vi "Resistance Test_BU3.vi"(0 "DMM ref in":refnum<visa-resource-name>, 2 "Resistance Test REF":refnum<vi>, 3 "Resistance Test Stop REF":refnum<vi>, 5 "DMM error in":errorcluster, 7 "Channel  Count":i32, 9 "ESP32 ref in":refnum<visa-resource-name>="COM4", 11 "ESP32 error in":errorcluster, 12 "Wait Current Stable Period":u32, 14 "Current Sense \nResitance Array":dbl[](array[numeric])) -> (1 "Array 2":bool[](array[boolean]), 6 "error?":bool, 8 "Array":dbl[](array[numeric]), 10 "ESP32 ref out":refnum<visa-resource-name>, 15 "ESP32 error out":errorcluster)   [LabVIEW 2023]
uses:
  <instrlib>/Agilent 3446X Series/Agilent 3446X Series.lvlib
panel:
  out "Array 3":i32[][](array[numeric])
  out "error? 2":bool
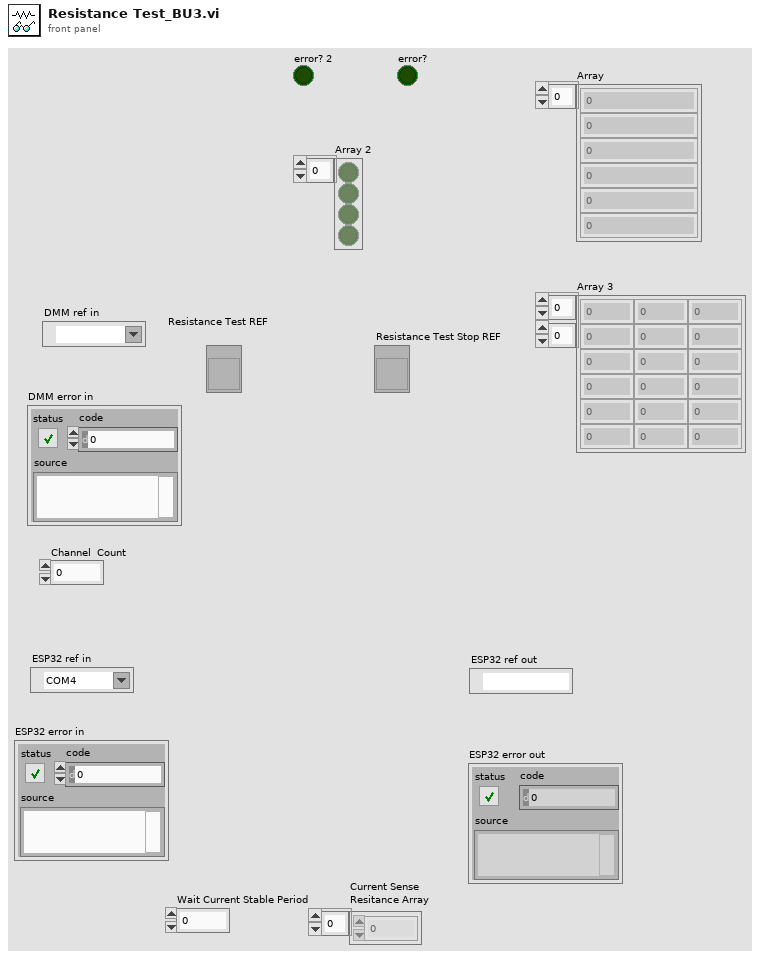
[diagram p1: front panel]
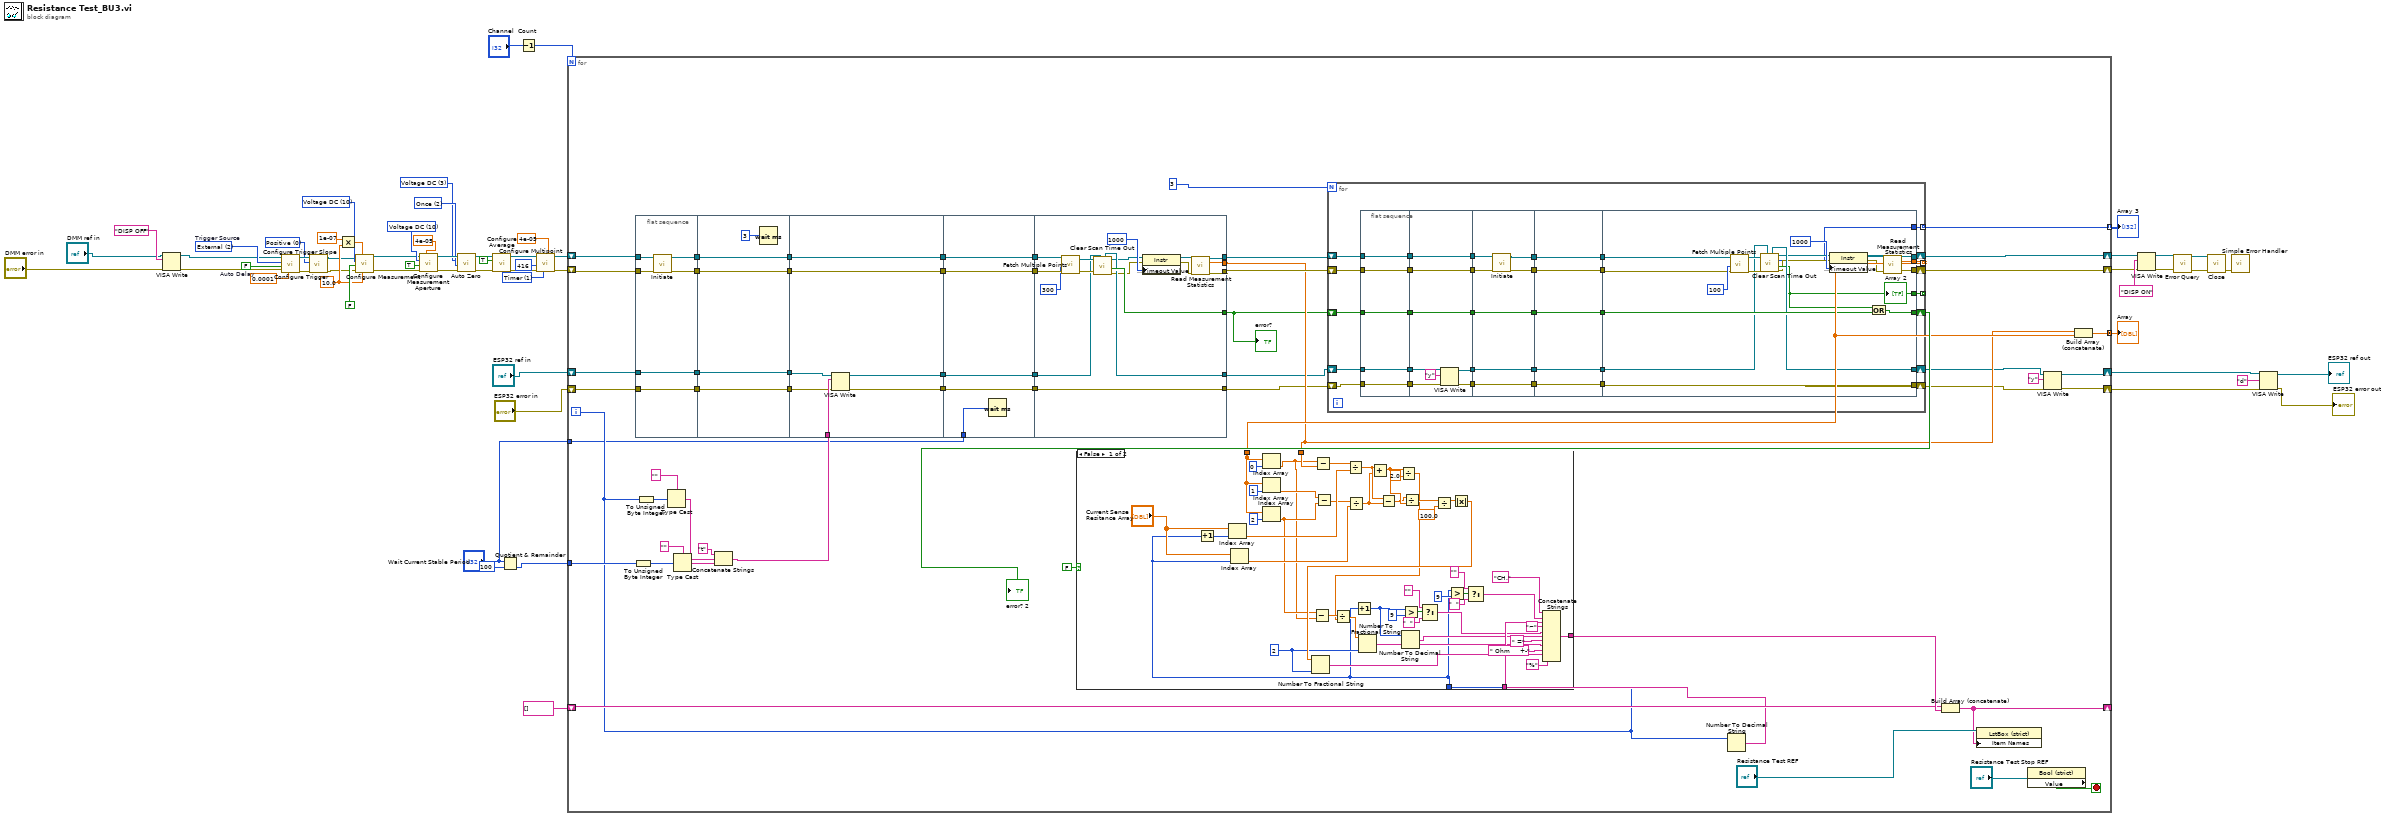
[diagram p0: block diagram]
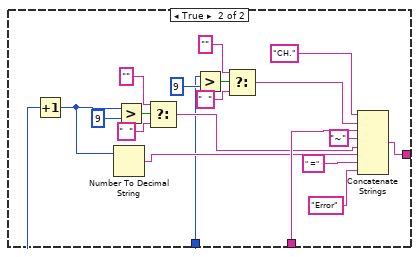
[diagram p2: hidden frame]
diagram:
  w20 = 0 items=["Positive", "Negative"] ("Trigger Edge (1: Negative)")
  w18 = 2 items=["Immediate", "Software (Bus)", "External"]  # Trigger Source
  w19 = FALSE  # Auto Delay
  w23 = 10.0 ("Manual Range (1)")
  w27 = 10 items=["Continuity", "Current AC", "Current DC", "Diode", "Frequency", "Resistance 4-wire", "Period", "Resistance 2-wire", "Temperature", "Voltage AC", "Voltage DC", "Voltage DC Ratio", "Capacitance"] ("Measurement Function (10: Voltage DC)")
  w31 = 1 items=["Immediate", "Timer"] ("Sample Source (0: Immediate)")
  w38 = 3 items=["Current DC", "Resistance", "Temperature", "Voltage DC"] ("Zero Type (0: Current DC)")
  w39 = 2 items=["Disable", "Enable", "Once"] ("Auto Zero (1: Enable)")
  w35 = 10 items=["Continuity", "Current AC", "Current DC", "Diode", "Frequency", "Resistance 4-wire", "Period", "Resistance 2-wire", "Temperature", "Voltage AC", "Voltage DC", "Voltage DC Ratio", "Capacitance"] ("Measurement Function (0: Continuity)")
  n1 = VISA Write(VISA resource name="DMM ref in", write buffer="DISP OFF", error in (no error)="DMM error in") -> (VISA resource name out=w2:refnum<visa-resource-name>, error out=w1:errorcluster)  [unwired: 1 out]
  n2 = call <instrlib>:"Configure Trigger.vi"("Manual Trigger Delay (1 s)"=0.0001, "error in (no error)"=w1, "Auto Delay (F:Disable)"=w19, "Trigger Source (0: Immediate)"=w18, "VISA resource name"=w2) -> ("error out"=w22:errorcluster, "VISA resource name out"=w21:refnum<visa-resource-name>)  [unwired: 1 in, 4 out]
  n3 = call <instrlib>:"Configure Trigger Slope.vi"("error in (no error)"=w22, "Trigger Edge (1: Negative)"=w20, "VISA resource name"=w21) -> ("error out"=w15:errorcluster, "VISA resource name out"=w16:refnum<visa-resource-name>)  [unwired: 7 in]
  n4 = Multiply(x=1e-07, y=w23) -> (x*y=w28:dbl)
  n5 = call <instrlib>:"Configure Measurement.vi"("Manual Range (1)"=w23, "Absolute Resolution (1E-6)"=w28, "error in (no error)"=w15, "Auto Range (T: Enable)"=FALSE, "Measurement Function (10: Voltage DC)"=w27, "VISA resource name"=w16) -> ("error out"=w24:errorcluster, "VISA resource name out"=w25:refnum<visa-resource-name>)  [unwired: 4 out]
  n6 = call <instrlib>:"Configure Measurement Aperture.vi"("Aperture Time (0.1s)"=4e-05, "error in (no error)"=w24, "Enable Aperture (F: Disable)"=TRUE, "Measurement Function (0: Continuity)"=w35, "VISA resource name"=w25) -> ("error out"=w42:errorcluster, "VISA resource name out"=w41:refnum<visa-resource-name>)  [unwired: 5 in]
  n7 = call <instrlib>:"Auto Zero.vi"("error in (no error)"=w42, "Auto Zero (1: Enable)"=w39, "Zero Type (0: Current DC)"=w38, "VISA resource name"=w41) -> ("error out"=w44:errorcluster, "VISA resource name out"=w43:refnum<visa-resource-name>)  [unwired: 6 in]
  n8 = call <instrlib>:"Configure Average.vi"("error in (no error)"=w44, "Enable Statistics (F: Disable)"=TRUE, "VISA resource name"=w43) -> ("error out"=w33:errorcluster, "VISA resource name out"=w34:refnum<visa-resource-name>)  [unwired: 7 in]
  n9 = Quotient & Remainder(x="Wait Current Stable Period", y=100) -> (floor(x/y)=w11:u32)  [unwired: 1 out]
  n10 = Decrement(x="Channel  Count") -> (x-1=w9:i32)
  n11 = call <instrlib>:"Configure Multipoint.vi"("Sample Interval (1 Second)"=4e-05, "Sample Source (0: Immediate)"=w31, "error in (no error)"=w33, "Sample Count (1)"=416, "VISA resource name"=w34) -> ("error out"=w13:errorcluster, "VISA resource name out"=w14:refnum<visa-resource-name>)  [unwired: 2 in, 3 out]
  n12 = for {
    N: w9 -> [_]
    shift-right: [w65] -> w46
    shift-left: "ESP32 ref in" -> [w100]
    shift-right: [w63] -> w10
    shift-left: "ESP32 error in" -> [w98]
    shift-right: [w110] -> w47
    shift-left: w13 -> [w104]
    shift-right: [w111] -> w48
    shift-left: w14 -> [w105]
    shift-right: [w113] -> _
    shift-left: string[] [] -> [w115]
    tunnel: w11 -> [w88]
    tunnel: [w81] -> w8 mode=concatenating
    tunnel: "Wait Current Stable Period" -> [w69]
    tunnel: [w61] -> w6 mode=indexing
    i -> [w85]
    stop <- w117 stop-if-true
    n13 = To Unsigned Byte Integer(number=w88) -> (unsigned 8bit integer=w92:u8)
    n14 = flat-sequence {
      tunnel: w104 -> [w190]
      tunnel: w105 -> [w192]
      tunnel: [w191] -> w109
      tunnel: [w189] -> w108
      tunnel: [w188] -> w101
      tunnel: w100 -> [w188]
      tunnel: w98 -> [w187]
      tunnel: [w187] -> w97
      tunnel: [w197] -> w107
      tunnel: [w196] -> w106
      tunnel: w109 -> [w197]
      tunnel: w108 -> [w196]
      tunnel: w101 -> [w194]
      tunnel: [w194] -> w99
      tunnel: w97 -> [w193]
      tunnel: [w193] -> w96
      tunnel: w107 -> [w204]
      tunnel: [w204] -> w75
      tunnel: w106 -> [w203]
      tunnel: [w203] -> w77
      tunnel: w99 -> [w202]
      tunnel: w96 -> [w200]
      tunnel: w87 -> [w201]
      tunnel: [w199] -> w73
      tunnel: [w198] -> w71
      tunnel: w77 -> [w209]
      tunnel: [w209] -> w76
      tunnel: w75 -> [w208]
      tunnel: [w208] -> w74
      tunnel: w73 -> [w207]
      tunnel: [w207] -> w72
      tunnel: w71 -> [w206]
      tunnel: [w206] -> w70
      tunnel: w69 -> [w205]
      tunnel: [w223] -> w102
      tunnel: [w224] -> w103
      tunnel: w76 -> [w226]
      tunnel: w74 -> [w225]
      tunnel: [w215] -> w78
      tunnel: w72 -> [w217]
      tunnel: [w221] -> w68
      tunnel: w70 -> [w221]
      tunnel: [w220] -> w82
      tunnel: [w216] -> w79
      frame #0 {
        n15 = call <instrlib>:"Initiate.vi"("error in (no error)"=w190, "VISA resource name"=w192) -> ("error out"=w189:errorcluster, "VISA resource name out"=w191:refnum<visa-resource-name>)  [unwired: 8 out]
      }
      frame #1 {
        n16 = Wait (ms)(milliseconds to wait=u32 3) -> ()  [unwired: 1 out]
      }
      frame #2 {
        n17 = VISA Write(VISA resource name=w202, write buffer=w201, error in (no error)=w200) -> (VISA resource name out=w199:refnum<visa-resource-name>, error out=w198:errorcluster)  [unwired: 1 out]
      }
      frame #3 {
        n18 = Wait (ms)(milliseconds to wait=w205) -> ()  [unwired: 1 out]
      }
      frame #4 {
        n19 = call <instrlib>:"Fetch Multiple Points.vi"("error in (no error)"=w226, "Timeout (10000 ms)"=300, "VISA resource name"=w225) -> ("error out"=w218:errorcluster, "VISA resource name out"=w219:refnum<visa-resource-name>)  [unwired: 1 in, 6 out]
        n20 = call "Clear Scan Time Out.vi"("ESP32 ref"=w217, "error in (no error)"=w218, "VISA Refnum in"=w219) -> ("error out"=w212:errorcluster, "error?"=w216:bool, "VISA Refnum out"=w213:refnum<visa-resource-name>, "ESP32 ref out"=w215:refnum<visa-resource-name>)  [unwired: 4 in, 1 out]
        n21 = property class="Instr"(reference=w213, error in=w212, "General Settings:Timeout Value"=u32 1000) -> (reference out=w211:refnum<visa-resource-name>, error out=w210:errorcluster)
        n22 = call <instrlib>:"Read Measurement Statistics.vi"("VISA resource name"=w211, "error in (no error)"=w210) -> ("VISA resource name out"=w224:refnum<visa-resource-name>, "Arithmetic Mean"=w220:dbl, "error out"=w223:errorcluster)  [unwired: 6 in, 5 out]
      }
    }
    n23 = To Unsigned Byte Integer(number=w85) -> (unsigned 8bit integer=w89:u8)
    n24 = Type Cast(type="" ("string"), x=w89) -> (*(type *) &x=w90:string)
    n25 = Type Cast(type="" ("string"), x=w92) -> (*(type *) &x=w91:string)
    n26 = Concatenate Strings("t" ("data in"), w90, w91) -> (w87:string)
    n27 = for {
      N: 3 -> [_]
      tunnel: [w257] -> w83 mode=indexing
      shift-right: [w256] -> w111
      shift-left: w103 -> [w259]
      shift-right: [w255] -> w110
      shift-left: w102 -> [w258]
      shift-right: [w253] -> w84
      shift-left: w79 -> [w254]
      tunnel: [w250] -> w80 mode=indexing
      shift-right: [w251] -> w66
      shift-left: w78 -> [w252]
      shift-right: [w248] -> w64
      shift-left: w68 -> [w249]
      tunnel: [w247] -> w61 mode=indexing
      n28 = flat-sequence {
        tunnel: w249 -> [w260]
        tunnel: w252 -> [w261]
        tunnel: w254 -> [w262]
        tunnel: w258 -> [w263]
        tunnel: w259 -> [w264]
        tunnel: [w264] -> w246
        tunnel: [w263] -> w245
        tunnel: [w262] -> w244
        tunnel: [w261] -> w243
        tunnel: [w260] -> w242
        tunnel: [w272] -> w241
        tunnel: [w271] -> w240
        tunnel: [w270] -> w239
        tunnel: [w268] -> w238
        tunnel: [w265] -> w237
        tunnel: w246 -> [w272]
        tunnel: w245 -> [w271]
        tunnel: w244 -> [w270]
        tunnel: w243 -> [w269]
        tunnel: w242 -> [w266]
        tunnel: w241 -> [w276]
        tunnel: w240 -> [w275]
        tunnel: [w274] -> w236
        tunnel: w239 -> [w279]
        tunnel: [w279] -> w234
        tunnel: w238 -> [w278]
        tunnel: [w278] -> w232
        tunnel: w237 -> [w277]
        tunnel: [w277] -> w230
        tunnel: [w273] -> w228
        tunnel: w236 -> [w284]
        tunnel: [w284] -> w235
        tunnel: w234 -> [w283]
        tunnel: [w283] -> w233
        tunnel: w232 -> [w282]
        tunnel: [w282] -> w231
        tunnel: w230 -> [w281]
        tunnel: [w281] -> w229
        tunnel: w228 -> [w280]
        tunnel: [w280] -> w227
        tunnel: [w304] -> w257
        tunnel: [w302] -> w256
        tunnel: [w301] -> w255
        tunnel: [w299] -> w253
        tunnel: [w295] -> w251
        tunnel: [w294] -> w250
        tunnel: w235 -> [w285]
        tunnel: w233 -> [w300]
        tunnel: w231 -> [w296]
        tunnel: w229 -> [w288]
        tunnel: [w288] -> w248
        tunnel: [w287] -> w247
        tunnel: w227 -> [w286]
        frame #0 {
        }
        frame #1 {
          n29 = VISA Write(VISA resource name=w269, write buffer="y", error in (no error)=w266) -> (VISA resource name out=w268:refnum<visa-resource-name>, error out=w265:errorcluster)  [unwired: 1 out]
        }
        frame #2 {
          n30 = call <instrlib>:"Initiate.vi"("error in (no error)"=w275, "VISA resource name"=w276) -> ("error out"=w274:errorcluster, "VISA resource name out"=w273:refnum<visa-resource-name>)  [unwired: 8 out]
        }
        frame #3 {
        }
        frame #4 {
          n31 = call <instrlib>:"Fetch Multiple Points.vi"("error in (no error)"=w285, "Timeout (10000 ms)"=100, "VISA resource name"=w286) -> ("error out"=w297:errorcluster, "VISA resource name out"=w298:refnum<visa-resource-name>)  [unwired: 1 in, 6 out]
          n32 = call "Clear Scan Time Out.vi"("ESP32 ref"=w296, "error in (no error)"=w297, "VISA Refnum in"=w298) -> ("error out"=w289:errorcluster, "error?"=w294:bool, "Time out count"=w287:i32, "VISA Refnum out"=w290:refnum<visa-resource-name>, "ESP32 ref out"=w295:refnum<visa-resource-name>)  [unwired: 4 in]
          n33 = property class="Instr"(reference=w290, error in=w289, "General Settings:Timeout Value"=u32 1000) -> (reference out=w292:refnum<visa-resource-name>, error out=w291:errorcluster)
          n34 = Or(x=w294, y=w300) -> (x .or. y?=w299:bool)
          n35 = call <instrlib>:"Read Measurement Statistics.vi"("VISA resource name"=w292, "error in (no error)"=w291) -> ("VISA resource name out"=w302:refnum<visa-resource-name>, "Arithmetic Mean"=w304:dbl, "error out"=w301:errorcluster)  [unwired: 6 in, 5 out]
        }
      }
    }
    "Array 2" <- w80
    "error? 2" <- w84
    n36 = Number To Decimal String(number=w85) -> (decimal integer string=w86:string)  [unwired: 1 in]
    n37 = case shown="False" FALSE {
      tunnel: [w162 w181] -> w116
      tunnel: w86 -> [w159 w178]
      tunnel: w83 -> [w147 _]
      tunnel: w85 -> [w123 w169]
      tunnel: w82 -> [w140 _]
      frame False {
        w131 = i16 2 ("precision (6)")
        n38 = Increment(x=w123) -> (x+1=w143:i32)
        n39 = Index Array(array="Current Sense \nResitance Array", index=w143) -> (element=w141:dbl)
        n40 = Index Array(array="Current Sense \nResitance Array", index=w123) -> (element=w138:dbl)
        n41 = Index Array(array=w147, index=0) -> (element=w127:dbl)
        n42 = Index Array(array=w147, index=1) -> (element=w128:dbl)
        n43 = Index Array(array=w147, index=2) -> (element=w129:dbl)
        n44 = Subtract(x=w129, y=w127) -> (x-y=w126:dbl)
        n45 = Subtract(x=w127, y=w140) -> (x-y=w144:dbl)
        n46 = Subtract(x=w128, y=w129) -> (x-y=w139:dbl)
        n47 = Divide(x=w144, y=w141) -> (x/y=w136:dbl)
        n48 = Divide(x=w139, y=w138) -> (x/y=w135:dbl)
        n49 = Increment(x=w123) -> (x+1=w152:i32)
        n50 = Add(x=w136, y=w135) -> (x+y=w122:dbl)
        n51 = Subtract(x=w136, y=w135) -> (x-y=w121:dbl)
        n52 = Divide(x=w122, y=2.0) -> (x/y=w125:dbl)
        n53 = Divide(x=w126, y=w125) -> (x/y=w124:dbl)
        n54 = Number To Fractional String(number=w124, precision (6)=w131) -> (F-format string=w133:string)  [unwired: 2 in]
        n55 = Number To Decimal String(number=w152) -> (decimal integer string=w151:string)  [unwired: 1 in]
        n56 = Greater?(x=w152, y=9) -> (0:w156:bool)
        n57 = Divide(x=w121, y=w122) -> (x/y=w134:dbl)
        n58 = Select(t="" ("string"), s=w156, f="  " ("string")) -> (s? t:f=w153:string)
        n59 = Divide(x=w134, y=100.0) -> (x/y=w120:dbl)
        n60 = Greater?(x=w123, y=9) -> (0:w165:bool)
        n61 = Absolute Value(x=w120) -> (abs(x)=w132:dbl)
        n62 = Number To Fractional String(number=w132, precision (6)=w131) -> (F-format string=w130:string)  [unwired: 2 in]
        n63 = Select(t="" ("string"), s=w165, f="  " ("string")) -> (s? t:f=w160:string)
        n64 = Concatenate Strings("CH." ("string"), w160, w159, "~" ("string"), w153, w151, " =" ("string"), w133, " Ohm     +-" ("string"), w130, "%" ("string")) -> (w162:string)
      }
      frame True {
        n65 = Increment(x=w169) -> (x+1=w171:i32)
        n66 = Number To Decimal String(number=w171) -> (decimal integer string=w170:string)  [unwired: 1 in]
        n67 = Greater?(x=w171, y=9) -> (0:w175:bool)
        n68 = Select(t="" ("string"), s=w175, f="  " ("string")) -> (s? t:f=w172:string)
        n69 = Greater?(x=w169, y=9) -> (0:w184:bool)
        n70 = Select(t="" ("string"), s=w184, f="  " ("string")) -> (s? t:f=w179:string)
        n71 = Concatenate Strings("CH." ("string"), w179, w178, "~" ("string"), w172, w170, " =" ("string"), "Error" ("string")) -> (w181:string)
      }
    }
    n72 = Build Array (concatenate)(w115, w116) -> (w113:string[])
    n73 = property class="LstBox (strict)"(reference="Resistance Test REF", "Item Names"=w113) -> ()  [unwired: 1 in, 2 out]
    n74 = property class="Bool (strict)"(reference="Resistance Test Stop REF") -> ("Value"=w117:bool)  [unwired: 1 in, 2 out]
    n75 = VISA Write(VISA resource name=w66, write buffer="y", error in (no error)=w64) -> (VISA resource name out=w65:refnum<visa-resource-name>, error out=w63:errorcluster)  [unwired: 1 out]
    n76 = Build Array (concatenate)(w82, w83) -> (w81:dbl[])
    "error?" <- w79
  }
  "Array" <- w8
  "Array 3" <- w6
  n77 = VISA Write(VISA resource name=w48, write buffer="DISP ON", error in (no error)=w47) -> (VISA resource name out=w55:refnum<visa-resource-name>, error out=w54:errorcluster)  [unwired: 1 out]
  n78 = call <instrlib>:"Error Query.vi"("error in (no error)"=w54, "VISA resource name"=w55) -> ("error out"=w60:errorcluster, "VISA resource name out"=w59:refnum<visa-resource-name>)  [unwired: 8 out]
  n79 = call <instrlib>:"Close.vi"("error in (no error)"=w60, "VISA resource name"=w59) -> ("error out"=w58:errorcluster)  [unwired: 9 out]
  n80 = call <vilib>:"Simple Error Handler.vi"("error in (no error)"=w58) -> ()  [unwired: 1 in, 8 out]
  n81 = VISA Write(VISA resource name=w46, write buffer="d" ("data in"), error in (no error)=w10) -> (VISA resource name out=→"ESP32 ref out":refnum<visa-resource-name>, error out=→"ESP32 error out":errorcluster)  [unwired: 1 out]
